vi "Set Current Limit.vi"(8 "error in (no error)":errorcluster, 10 "Current Limit (A)":dbl, 11 "NI_PSU in":refnum<class "NI_PSU.lvclass">) -> (0 "error out":errorcluster, 3 "NI_PSU out":refnum<class "NI_PSU.lvclass">)   [LabVIEW 2024, in "HAL_Example.lvlib" / "NI_PSU.lvclass"]
uses:
  NI_PSU.lvclass
  PSU/PSU.lvclass
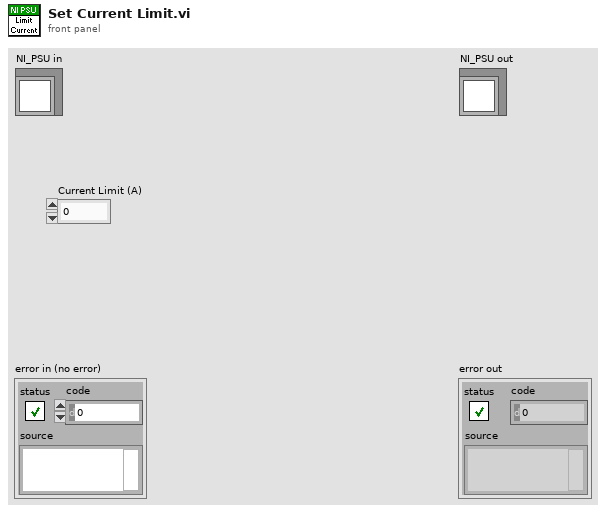
[diagram p1: front panel]
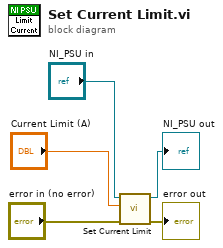
[diagram p0: block diagram]
diagram:
  n1 = call-parent "Set Current Limit.vi"("error in (no error)"="error in (no error)", "Current Limit (A)"="Current Limit (A)", "PSU in"="NI_PSU in") -> ("error out"=→"error out":errorcluster, "PSU out"=→"NI_PSU out":refnum<class "NI_PSU.lvclass">)  [unwired: 7 in]
